vi "ws_read GET parameters.vi"(2 "httpRequestID":u32) -> (0 "GET query params":T1)   [LabVIEW 2011]
doc: "Returns the parameters that a CGI request contains. If the request contains a single parameter, the calling VI must use <B>query string</B>. If the request contains a list of parameters, the calling VI must use <B>query params</B>."
uses:
  <vilib>/addons/internet/utils/keyedarr.llb/Keyed Array.ctl
  <vilib>/wsapi/NI_WebServices.lvlib
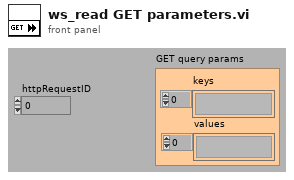
[diagram p1: front panel]
types:
  T1 = typedef "Keyed Array.ctl" = cluster{"keys":string[], "values":string[]}
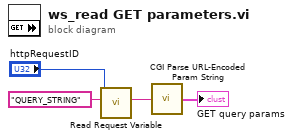
[diagram p0: block diagram]
diagram:
  n1 = call <vilib>:"Read Request Variable.vi"("variable name"="QUERY_STRING", "httpRequestID"="httpRequestID") -> ("value"=w1:string)  [unwired: 7 in, 2 out]
  n2 = call <vilib>:"CGI Parse URL-Encoded Param String.vi"("url-encoded param string"=w1) -> ("params"=→"GET query params":T1)
